vi "Get SDK3Handle.vi"(11 "Handle":i32) -> (2 "function return":u32, 3 "Handle out":i32)   [LabVIEW 2018, in "AndorSDK.lvlib"]
doc: "EXPNETTYPE unsigned int WINAPI GetSDK3Handle(int * Handle);"
uses:
  AndorSDK.lvlib
  ATMCD32D.dll
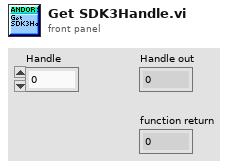
[diagram p1: front panel]
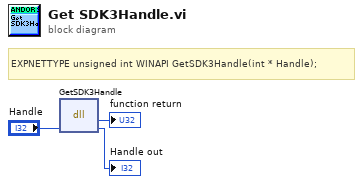
[diagram p0: block diagram]
diagram:
  # "EXPNETTYPE unsigned int WINAPI GetSDK3Handle(int * Handle);"
  n1 = dll-call lib="PTH2babs E\nPersönliches02 - Arbeit03-HiwijobsLabviewCodelibANDOR\tAndor SDK\nATMCD32D.*" fn="GetSDK3Handle"("Handle"="Handle") -> (→"function return":u32, "Handle"=→"Handle out":i32)  [unwired: 3 in, 2 out]
